vi "DELETEList Controls.vi"(8 "error in (no error)":errorcluster, 11 "Rename in":refnum<class "ProjectItem.lvclass">) -> (0 "error out":errorcluster, 3 "Rename out":refnum<class "ProjectItem.lvclass">)   [LabVIEW 2019]
uses:
  <vilib>/regexp/Match Regular Expression.xnode
  <vilib>/Utility/traverseref.llb/VI Scripting - Traverse.lvlib
  ProjectItem.lvclass
  <vilib>/LabVIEW Icon API/lv_icon/Classes/Icon/Icon.lvclass
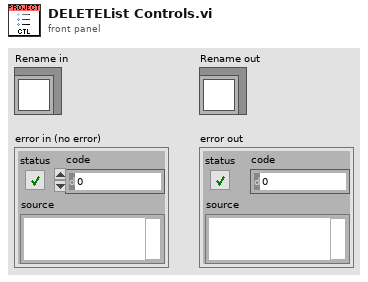
[diagram p1: front panel]
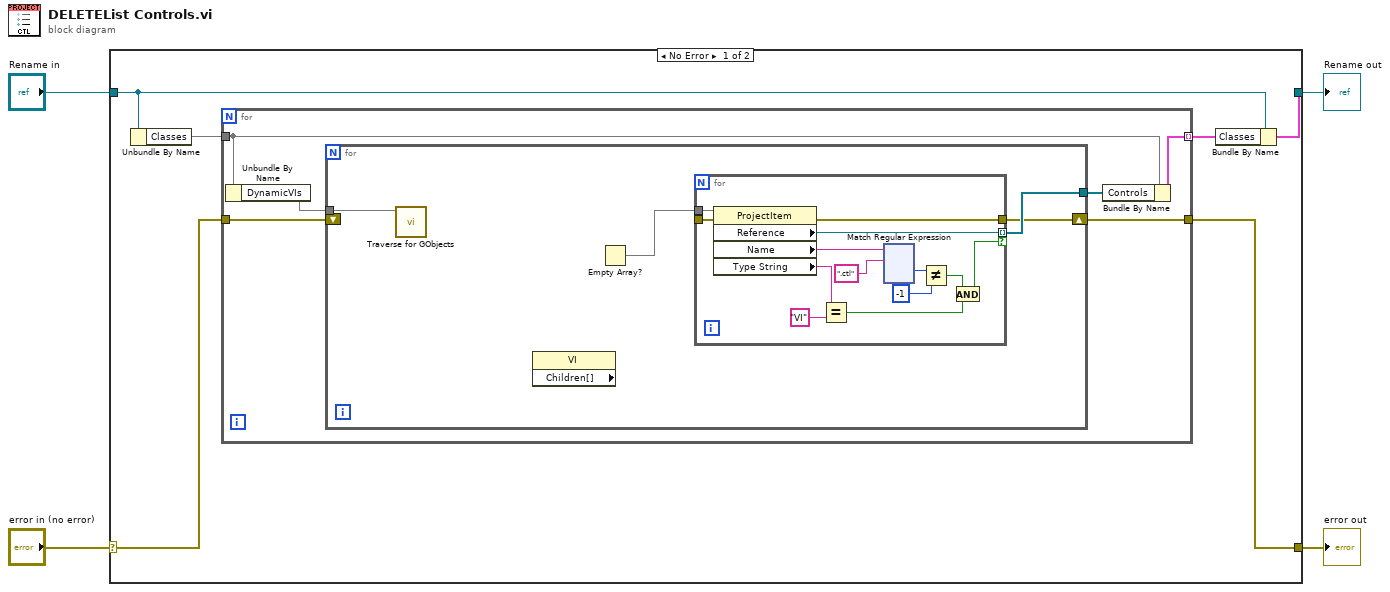
[diagram p0: block diagram]
diagram:
  n1 = case shown="No Error" "error in (no error)" {
    selector: "error in (no error)" -> [w6 w150]
    tunnel: [w9 w149] -> w4
    tunnel: "Rename in" -> [w8 w149]
    tunnel: [w5 w150] -> w2
    frame No Error {
      n2 = Unbundle By Name(w8) -> ("Classes"=w7)
      n3 = for {
        tunnel: w7 -> [w16]
        tunnel: w6 -> [w12]
        tunnel: [w11] -> w5
        tunnel: [w15] -> w10 mode=indexing
        n4 = Unbundle By Name(w16) -> ("DynamicVIs"=w14)
        n5 = for {
          tunnel: w14 -> [w17]
          tunnel: [w20] -> w13
          shift-right: [w18] -> w11
          shift-left: w12 -> [_]
          n6 = call <vilib>:"Traverse for GObjects.vi"("VI Refnum"=w17) -> ()  [unwired: 7 in, 4 out]
          n7 = property class="VI" props=["Children[]"]() -> ()  [unwired: 2 in, 3 out]
          n8 = for {
            tunnel: [w34] -> w21
            tunnel: [w29] -> w20 mode=indexing if=w26
            tunnel: [w28] -> w19
            tunnel: [w27] -> w18
            n9 = property class="ProjectItem"(reference=w34, error in=w28) -> (error out=w27:errorcluster, "Reference"=w29:refnum<vi>, "Name"=w33:string, "Type String"=w25:string)  [unwired: 1 out]
            n10 = Equal?(x=w25, y="VI") -> (x = y?=w23:bool)
            n11 = xnode "Match Regular Expression"("input string"=w33, "regular expression"=".ctl") -> ("offset past match"=w31:i32)  [unwired: 4 in, 4 out]
            n12 = Not Equal?(x=w31, y=-1) -> (x != y?=w22:bool)
            n13 = And(x=w22, y=w23) -> (x .and. y?=w26:bool)
          }
          n14 = Empty Array?(array=w21) -> ()  [unwired: 1 out]
        }
        n15 = Bundle By Name(cluster=w16, "Controls"=w13) -> (w15:cluster{})
      }
      n16 = Bundle By Name(cluster=w8, "Classes"=w10) -> (w9:cluster{})
    }
    frame Error {
    }
  }
  "Rename out" <- w4
  "error out" <- w2
